vi "Rodrigues vector.vi"(10 "R Rotation Matrix":T1 format="%#_6f") -> (2 "Rodrigues vector":dbl[](array[numeric]))   [LabVIEW 2025]
uses:
  <vilib>/Analysis/Matrix/Datatypes/RealMatrix.ctl
  <vilib>/Analysis/_algsub.llb/Real Matrix Trace.vi
  <vilib>/Analysis/NI_AALPro.lvlib
  <vilib>/Analysis/Matrix/NI_Matrix.lvlib
panel:
  out "rvec_x":dbl
  out "rvec_y":dbl
  out "rvec_z":dbl
  out "kz":dbl
  out "ky":dbl
  out "kx":dbl
  out "s":dbl
  out "Angle (rad)":dbl
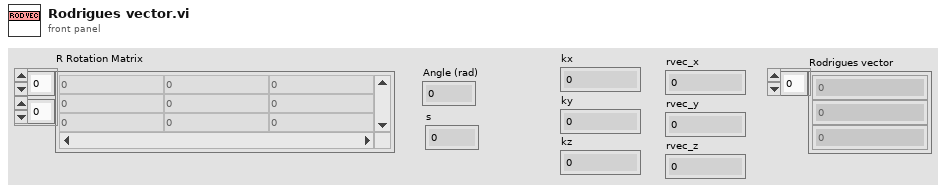
[diagram p1: front panel]
types:
  T1 = typedef "NI_Matrix.lvlib/RealMatrix.ctl" = dbl[][]
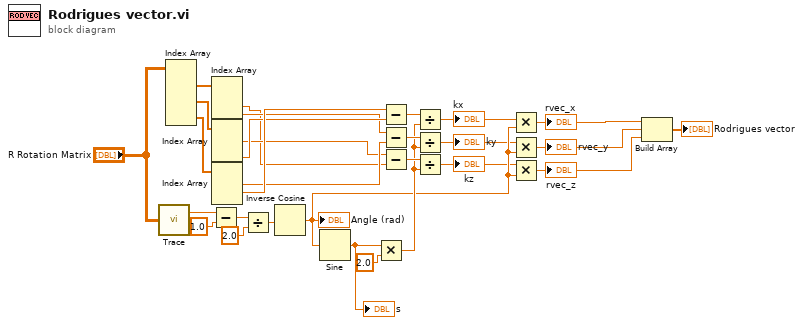
[diagram p0: block diagram]
diagram:
  n1 = call-poly <vilib>:"Trace.vi"("Input Matrix"="R Rotation Matrix") -> ("trace"=w29:dbl)  [unwired: 1 out]
  n2 = Index Array(array="R Rotation Matrix") -> (element #1=w23:dbl[], element #2=w22:dbl[], element #3=w21:dbl[])  [unwired: 6 in]
  n3 = Subtract(x=w29, y=1.0) -> (x-y=w27:dbl)
  n4 = Index Array(array=w23) -> (element #2=w10:dbl, element #3=w14:dbl)  [unwired: 3 in, 1 out]
  n5 = Index Array(array=w22) -> (element #1=w11:dbl, element #3=w19:dbl)  [unwired: 3 in, 1 out]
  n6 = Index Array(array=w21) -> (element #1=w13:dbl, element #2=w20:dbl)  [unwired: 3 in, 1 out]
  n7 = Divide(x=w27, y=2.0) -> (x/y=w25:dbl)
  n8 = Inverse Cosine(1:w25) -> (0:w7:dbl)
  "Angle (rad)" <- w7
  n9 = Sine(x=w7) -> (sin(x)=w16:dbl)
  "s" <- w16
  n10 = Multiply(x=w16, y=2.0 ("x")) -> (x*y=w9:dbl)
  n11 = Subtract(x=w20, y=w19) -> (x-y=w18:dbl)
  n12 = Subtract(x=w14, y=w13) -> (x-y=w15:dbl)
  n13 = Subtract(x=w11, y=w10) -> (x-y=w12:dbl)
  n14 = Divide(x=w18, y=w9) -> (x/y=w8:dbl)
  "kx" <- w8
  n15 = Divide(x=w15, y=w9) -> (x/y=w6:dbl)
  "ky" <- w6
  n16 = Divide(x=w12, y=w9) -> (x/y=w5:dbl)
  "kz" <- w5
  n17 = Multiply(x=w8, y=w7) -> (x*y=w4:dbl)
  "rvec_x" <- w4
  n18 = Multiply(x=w6, y=w7) -> (x*y=w3:dbl)
  "rvec_y" <- w3
  n19 = Multiply(x=w5, y=w7) -> (x*y=w2:dbl)
  "rvec_z" <- w2
  n20 = Build Array(w4, w3, w2) -> (→"Rodrigues vector":dbl[])
